vi "ROLFPython.vi"() -> ()   [LabVIEW 2019]
panel:
  out "data string 1":string
  out "data string 2":string
  out "data string 3":string
  out "data string 4":string
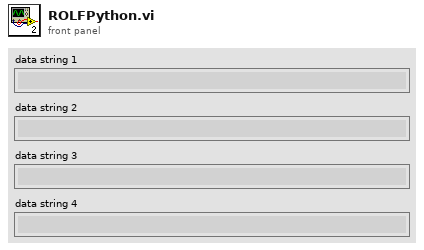
[diagram p1: front panel]
types:
  T1 = enum16{"big-endian, network order", "native, host order", "little-endian"}
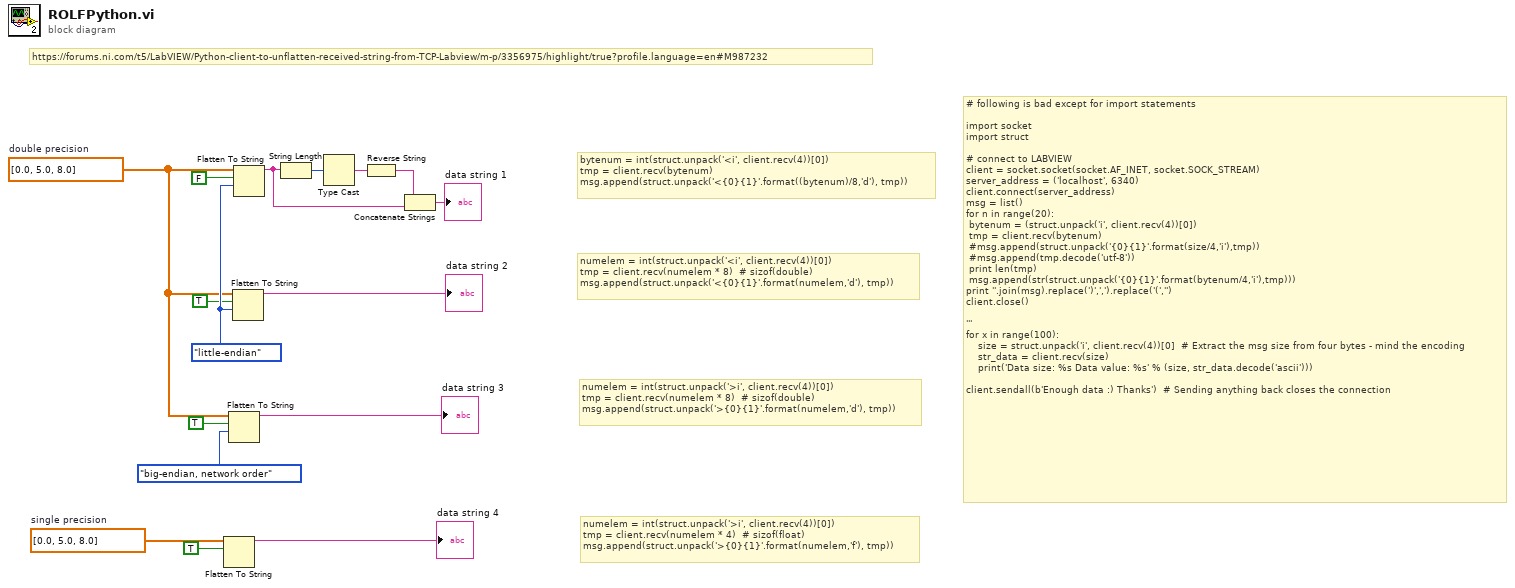
[diagram p0: block diagram]
diagram:
  w1 = sgl[] [0.0, 5.0, 8.0]  # single precision
  w4 = dbl[] [0.0, 5.0, 8.0]  # double precision
  w10 = T1."little-endian" ("byte order (0:big-endian, network order)")
  # "# following is bad except for import statements\n\nimport socket\nimport struct\n\n# connect to LABVIEW\nclient = socket.socket(socket.AF_INET, socket.SOCK_STREAM)\nserver_address = ('localhost', 6340)\nclient.connect(server_address)\nmsg = list()\nfor n in range(20):\n\tbytenum = (struct.unpack('i', client.recv(4))[0])\n\ttmp = client.recv(bytenum)\n\t#msg.append(struct.unpack('{0}{1}'.format(size/4,'i'),tmp))\n\t#msg.append(tmp.decode('utf-8'))\n\tprint len(tmp)\n\tmsg.append(str(struct.unpack('{0}{1}'.format(bytenum/4,'i'),tmp)))\nprint ''.join(msg).replace(')',',').replace('(','')\nclient.close()\n\n'''\nfor x in range(100):\n    size = struct.unpack('i', client.recv(4))[0]  # Extract the msg size from four bytes - mind the encoding\n    str_data = client.recv(size)\n    print('Data size: %s Data value: %s' % (size, str_data.decode('ascii')))\n\nclient.sendall(b'Enough data :) Thanks')  # Sending anything back closes the connection"
  # "https://forums.ni.com/t5/LabVIEW/Python-client-to-unflatten-received-string-from-TCP-Labview/m-p/3356975/highlight/true?profile.language=en#M987232"
  # "numelem = int(struct.unpack('>i', client.recv(4))[0])\ntmp = client.recv(numelem * 4)  # sizof(float)\nmsg.append(struct.unpack('>{0}{1}'.format(numelem,'f'), tmp))"
  # "numelem = int(struct.unpack('>i', client.recv(4))[0])\ntmp = client.recv(numelem * 8)  # sizof(double)\nmsg.append(struct.unpack('>{0}{1}'.format(numelem,'d'), tmp))"
  # "numelem = int(struct.unpack('<i', client.recv(4))[0])\ntmp = client.recv(numelem * 8)  # sizof(double)\nmsg.append(struct.unpack('<{0}{1}'.format(numelem,'d'), tmp))"
  # "bytenum = int(struct.unpack('<i', client.recv(4))[0])\ntmp = client.recv(bytenum)\nmsg.append(struct.unpack('<{0}{1}'.format((bytenum)/8,'d'), tmp))"
  n1 = Flatten To String(anything=w1, prepend array or string size? (T)=TRUE) -> (data string=→"data string 4":string)  [unwired: 2 in, 2 out]
  n2 = Flatten To String(anything=w4, prepend array or string size? (T)=TRUE, byte order (0:big-endian, network order)=T1."big-endian, network order") -> (data string=→"data string 3":string)  [unwired: 1 in, 2 out]
  n3 = Flatten To String(anything=w4, prepend array or string size? (T)=TRUE, byte order (0:big-endian, network order)=w10) -> (data string=→"data string 2":string)  [unwired: 1 in, 2 out]
  n4 = Flatten To String(anything=w4, prepend array or string size? (T)=FALSE, byte order (0:big-endian, network order)=w10) -> (data string=w12:string)  [unwired: 1 in, 2 out]
  n5 = String Length(string=w12) -> (length=w15:i32)
  n6 = Type Cast(x=w15) -> (*(type *) &x=w14:string)  [unwired: 1 out]
  n7 = Reverse String(1:w14) -> (0:w13:string)
  n8 = Concatenate Strings(w13, w12) -> (→"data string 1":string)
